vi "addDelayTicks.vi"(8 "error in (no error)":errorcluster, 10 "Ticks":u16, 11 "Modbus in":refnum<class "Modbus.lvclass">) -> (0 "error out":errorcluster, 3 "Modbus out":refnum<class "Modbus.lvclass">)   [LabVIEW 2016, in "RTModbus.lvlib" / "Modbus.lvclass"]
uses:
  Modbus.lvclass
  DataTypes/Frame.ctl
  RTModbus.lvlib
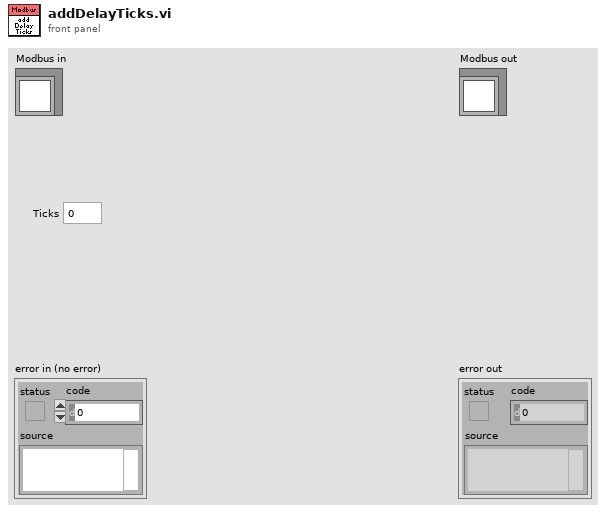
[diagram p1: front panel]
types:
  T1 = typedef "RTModbus.lvlib/Frame.ctl" = cluster{"Data":u8[], "WaitForTrigger":bool, "WaitForRx":u16, "TriggerIRQ":bool, "DelayTicks":u16, "DelayMicroseconds":u16, "DelayMilliseconds":u16}
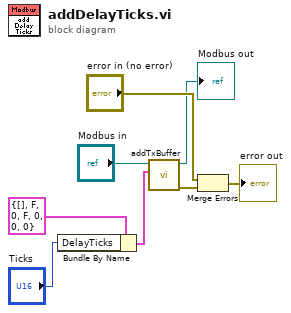
[diagram p0: block diagram]
diagram:
  n1 = Bundle By Name(cluster=T1 {"Data"=[], "WaitForTrigger"=FALSE, "WaitForRx"=0, "TriggerIRQ"=FALSE, "DelayTicks"=0, "DelayMicroseconds"=0, "DelayMilliseconds"=0} ("Frame"), "DelayTicks"="Ticks") -> (w6:T1)
  n2 = call-dynamic "addTxBuffer.vi"("Frame"=w6, "Modbus in"="Modbus in") -> ("error out"=w4:errorcluster, "Modbus out"=→"Modbus out":refnum<class "Modbus.lvclass">)  [unwired: 8 in]
  n3 = Merge Errors("error in (no error)", w4) -> (→"error out":errorcluster)
